vi "InitWaferArea.vi"(1 "Strings []":string[](array[string]), 2 "MeasureCntl":refnum<vi>) -> ()   [LabVIEW 2012]
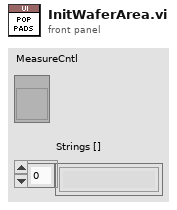
[diagram p1: front panel]
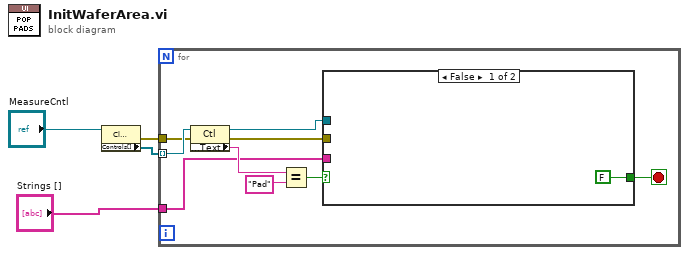
[diagram p0: block diagram]
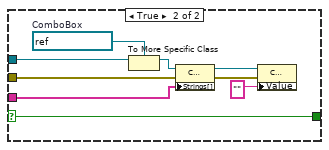
[diagram p2: hidden frame]
diagram:
  n1 = property class="Clust (strict)"(reference="MeasureCntl") -> (error out=w1:errorcluster, "Controls[]"=w3:refnum<vi>[])  [unwired: 1 in, 1 out]
  n2 = for {
    tunnel: w3 -> [w13] mode=indexing
    tunnel: "Strings []" -> [w8]
    tunnel: w1 -> [w6]
    stop <- w5 stop-if-true
    n3 = property class="Ctl"(reference=w13, error in=w6) -> (reference out=w9:refnum<vi>, error out=w7:errorcluster, "Label.Text"=w12:string)
    n4 = Equal?(x=w12, y="Pad") -> (x = y?=w10:bool)
    n5 = case shown="False" w10 {
      selector: w10 -> [_ w15]
      tunnel: w9 -> [_ w23]
      tunnel: w8 -> [_ w20]
      tunnel: w7 -> [_ w16]
      tunnel: [FALSE w15] -> w5
      frame False {
      }
      frame True {
        w22 = refnum<vi> refnum  # ComboBox
        n6 = To More Specific Class(target class=w22, reference=w23) -> (specific class reference=w21:refnum<vi>)  [unwired: 1 in, 1 out]
        n7 = property class="CmbBox"(reference=w21, error in=w16, "Strings[]"=w20) -> (reference out=w19:refnum<vi>, error out=w17:errorcluster)
        n8 = property class="CmbBox"(reference=w19, error in=w17, "Value"="") -> ()  [unwired: 2 out]
      }
    }
  }
